vi "ManagementRandomData.vi"(8 "error in (no error)":errorcluster, 11 "DataFlowIN":T1) -> (0 "error out":errorcluster, 3 "DataFlowOUT":T1)   [LabVIEW 2017]
doc: "Subpanel Plugin VI that displays a random value, multiplied by a user-specified value, in a waveform chart."
uses:
  classes/DataCollector.lvclass
  classes/DataHandler.lvclass
  classes/SimulationParameter.lvclass
panel:
  out "Random Number Chart":dbl(graph)
  in  "Multiplier":dbl(slide)=2.0 scale=0.0..10.0
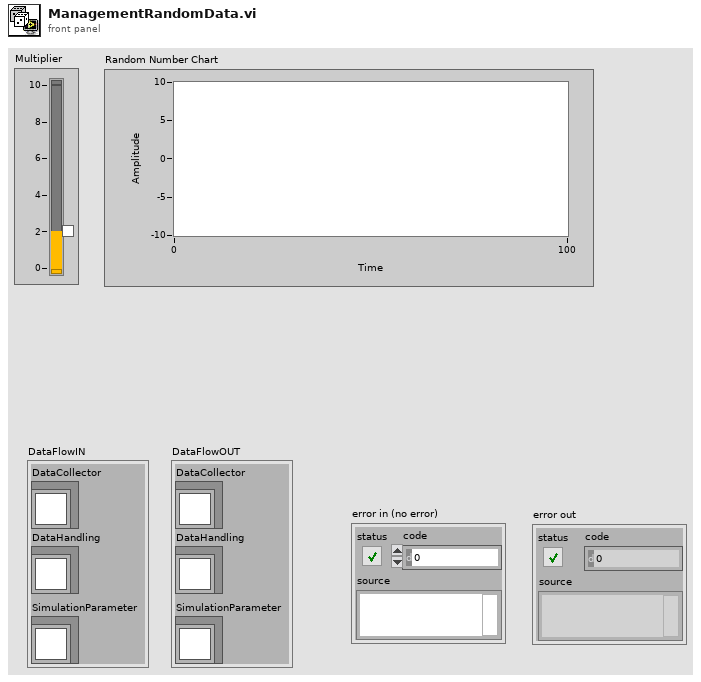
[diagram p1: front panel]
types:
  T1 = cluster{"DataCollector":refnum<class "DataCollector.lvclass">, "DataHandling":refnum<class "DataHandler.lvclass">, "SimulationParameter":refnum<class "SimulationParameter.lvclass">}
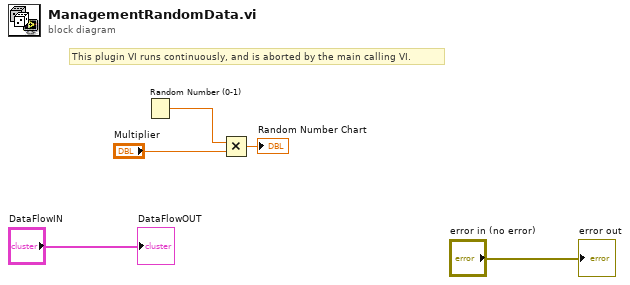
[diagram p0: block diagram]
diagram:
  # "This plugin VI runs continuously, and is aborted by the main calling VI."
  n1 = Random Number (0-1)() -> (number: 0 to 1=w3:dbl)
  n2 = Multiply(x=w3, y="Multiplier") -> (x*y=→"Random Number Chart":dbl)
  "error out" <- "error in (no error)"
  "DataFlowOUT" <- "DataFlowIN"
